vi "LabS6_Algoritmo1.vi"() -> ()   [LabVIEW 2012]
uses:
  <vilib>/Analysis/_algsub.llb/Real Vector Norm.vi
  <vilib>/Analysis/baseanly.llb/Real Dot Product.vi
  <vilib>/Analysis/NI_AALBase.lvlib
  <vilib>/Analysis/NI_AALPro.lvlib
panel:
  out "error":dbl=-7.601211530344765e-08
  out "norma":dbl=0.21066048226108744
  out "Chart Signal":cluster{"X * Y":dbl, "X * Y":dbl}(graph)={"X * Y"=0.030176439232253, "X * Y"=0.030176515244368304}
  out "W(k+1)":dbl[](array[numeric])=[0.9999995977283248, 0.10000036055977748]
  out "Chart Error":dbl(graph)=-7.601211530344765e-08
  in  "alpha":dbl=0.05
  in  "b":dbl[](array[numeric])=[1.0, 0.1]
  in  "Offset":dbl
  in  "A":dbl=1.0
  out "T":dbl=0.01
  in  "Fcon":dbl(knob)=3.229536374351221 scale=1.0..20.0
  in  "Fs":dbl=100.0
  in  "Tfinal":dbl=1000.0
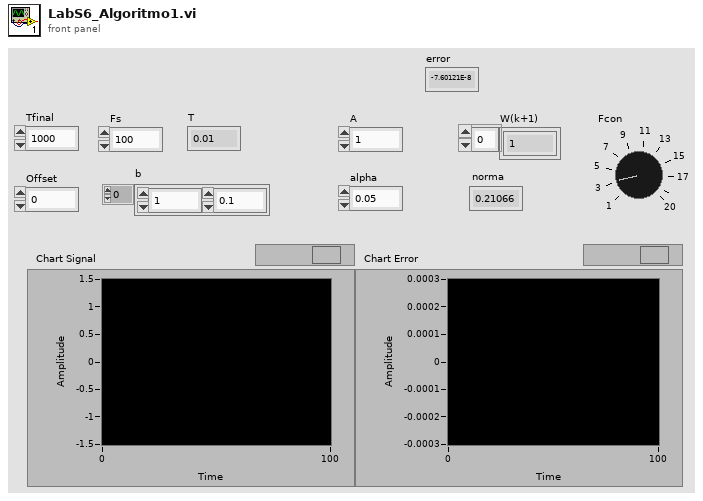
[diagram p1: front panel]
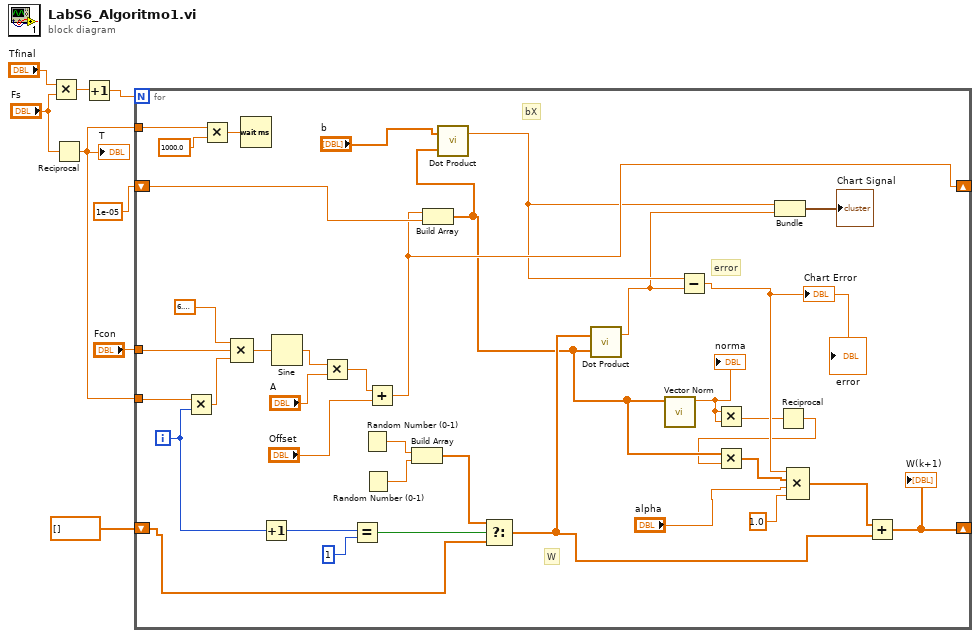
[diagram p0: block diagram]
diagram:
  n1 = Multiply(x="Tfinal", y="Fs") -> (x*y=w7:dbl)
  n2 = Reciprocal(x="Fs") -> (1/x=w1:dbl)
  "T" <- w1
  n3 = Increment(x=w7) -> (x+1=w6:dbl)
  n4 = for {
    N: w6 -> [_]
    tunnel: w1 -> [w43]
    tunnel: "Fcon" -> [w44]
    shift-right: [w22] -> _
    shift-left: 1e-05 ("element") -> [w28]
    shift-right: [w23] -> _
    shift-left: dbl[] [] -> [w18]
    tunnel: w1 -> [w16]
    i -> [w35]
    # "W"
    # "bX"
    # "error"
    n5 = Multiply(x=w43, y=w35) -> (x*y=w42:dbl)
    n6 = Multiply(x=w16, y=1000.0) -> (x*y=w17:dbl)
    n7 = Compound Arithmetic op=MULTIPLY(6.283185307179586, w44, w42) -> (w41:dbl)
    n8 = Wait (ms)(milliseconds to wait=w17) -> ()  [unwired: 1 out]
    n9 = Increment(x=w35) -> (x+1=w34:i32)
    n10 = Sine(x=w41) -> (sin(x)=w40:dbl)
    n11 = Multiply(x=w40, y="A") -> (x*y=w38:dbl)
    n12 = Equal?(x=w34, y=1) -> (x = y?=w32:bool)
    n13 = Random Number (0-1)() -> (number: 0 to 1=w31:dbl)
    n14 = Random Number (0-1)() -> (number: 0 to 1=w30:dbl)
    n15 = Add(x=w38, y="Offset") -> (x+y=w22:dbl)
    n16 = Build Array(w31, w30) -> (w29:dbl[])
    n17 = Build Array(w22, w28) -> (w11:dbl[])
    n18 = call-poly <vilib>:"Dot Product.vi"("Y Vector"=w11, "X Vector"="b") -> ("X * Y"=w21:dbl)  [unwired: 1 out]
    n19 = Select(t=w29, s=w32, f=w18) -> (s? t:f=w25:dbl[])
    n20 = call-poly <vilib>:"Dot Product.vi"("Y Vector"=w11, "X Vector"=w25) -> ("X * Y"=w20:dbl)  [unwired: 1 out]
    n21 = call-poly <vilib>:"Vector Norm.vi"("Input Vector"=w11) -> ("norm"=w13:dbl)  [unwired: 9 in, 1 out]
    "norma" <- w13
    n22 = Subtract(x=w21, y=w20) -> (x-y=w19:dbl)
    "Chart Error" <- w19
    "error" <- w19
    n23 = Multiply(x=w13, y=w13) -> (x*y=w12:dbl)
    n24 = Bundle("X * Y"=w21, "X * Y"=w20) -> (→"Chart Signal":cluster{"X * Y":dbl, "X * Y":dbl})  [unwired: 1 in]
    n25 = Reciprocal(x=w12) -> (1/x=w10:dbl)
    n26 = Multiply(x=w11, y=w10) -> (x*y=w9:dbl[])
    n27 = Compound Arithmetic op=MULTIPLY(w19, w9, "alpha", 1.0 ("value")) -> (w24:dbl[])
    n28 = Add(x=w24, y=w25) -> (x+y=w23:dbl[])
    "W(k+1)" <- w23
  }
